vi "Tree Create.vi"(8 "error in (no error)":errorcluster, 9 "Mode (Normal)":T1, 10 "Shot":i32, 11 "Name":string) -> (0 "error out":errorcluster, 3 "Tree DVR out":refnum<data-value>)   [LabVIEW 2015, in "MDSplus.lvlib"]
uses:
  <vilib>/MDSplus/Library/MDSplus.lvlib
  <vilib>/MDSplus/Classes/Tree_Class/Tree.lvclass
  <vilib>/MDSplus/Library/Tree/Tree Open Mode.ctl
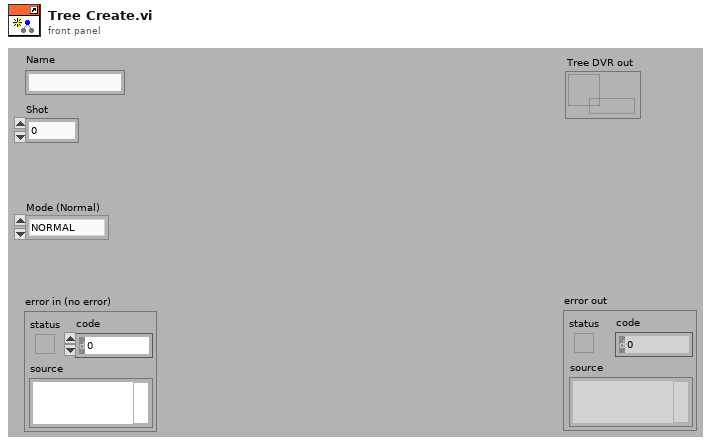
[diagram p1: front panel]
types:
  T1 = typedef "MDSplus.lvlib/Tree Open Mode.ctl" = enum16{"NORMAL", "EDIT", "NEW", "READONLY"}
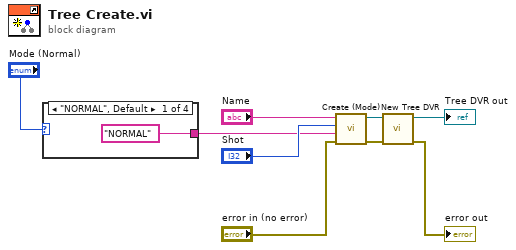
[diagram p0: block diagram]
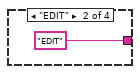
[diagram p2: hidden frame]
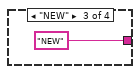
[diagram p3: hidden frame]
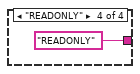
[diagram p4: hidden frame]
diagram:
  n1 = case shown="\"NORMAL\", Default" "Mode (Normal)" {
    tunnel: ["NORMAL" "EDIT" "NEW" "READONLY"] -> w1
    frame "NORMAL", Default {
    }
    frame "EDIT" {
    }
    frame "NEW" {
    }
    frame "READONLY" {
    }
  }
  n2 = call <vilib>:"Create (Mode).vi"("error in (no error)"="error in (no error)", "Mode"=w1, "Shot"="Shot", "Name"="Name") -> ("error out"=w7:errorcluster, "Tree out"=w8:refnum<class "Tree.lvclass">)  [unwired: 6 in]
  n3 = call <vilib>:"New Tree DVR.vi"("error in (no error)"=w7, "Tree in"=w8) -> ("error out"=→"error out":errorcluster, "Tree DVR out"=→"Tree DVR out":refnum<data-value>)  [unwired: 8 in]
